vi "AxisWriteRegs.vi"(8 "error in":errorcluster, 10 "AxisWriteValues":T1={"AxisTarget"=0.0, "AxisTargetVel"=1.0, "AxisStartReq"=FALSE, "AxisStopReq"=FALSE, "AxisClearReq"=FALSE, "AxisMovetype"=FALSE, "AxisMotorON"=FALSE, "MoveModeControl"=0, "AxisHomingVel"=1.0, "AxisAccDecc"=30.0} {"MoveModeControl" items=["Absolute"=1, "Relative"=2, "Velocity"=3, "Homing"=4, "none"=0]}, 11 "Modbus master":refnum<class "Modbus Master.lvclass">) -> (0 "error out":errorcluster)   [LabVIEW 2020, in "SMCD14_lib.lvlib"]
uses:
  SMCD14_lib.lvlib
  <vilib>/Modbus/master/Modbus Master.lvclass
  AxisWriteValues_typedef.ctl
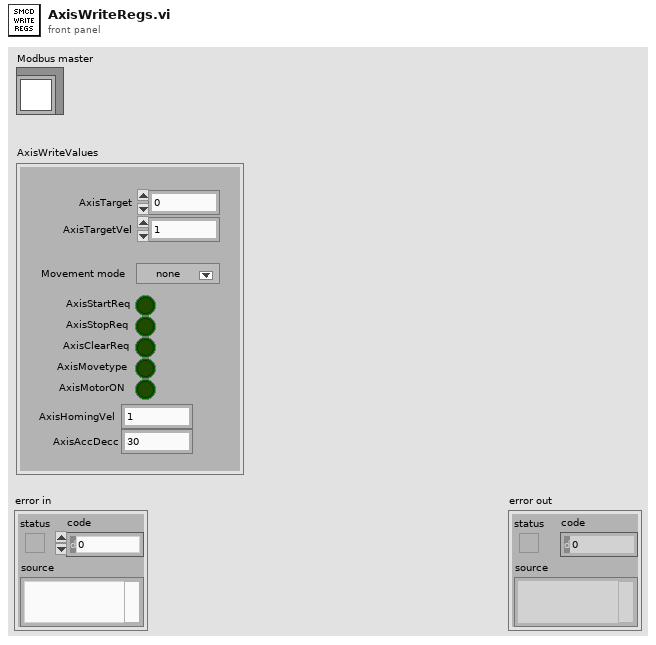
[diagram p1: front panel]
types:
  T1 = typedef "SMCD14_lib.lvlib/AxisWriteValues_typedef.ctl" = cluster{"AxisTarget":dbl, "AxisTargetVel":dbl, "AxisStartReq":bool, "AxisStopReq":bool, "AxisClearReq":bool, "AxisMovetype":bool, "AxisMotorON":bool, "MoveModeControl":u16, "AxisHomingVel":dbl, "AxisAccDecc":dbl}
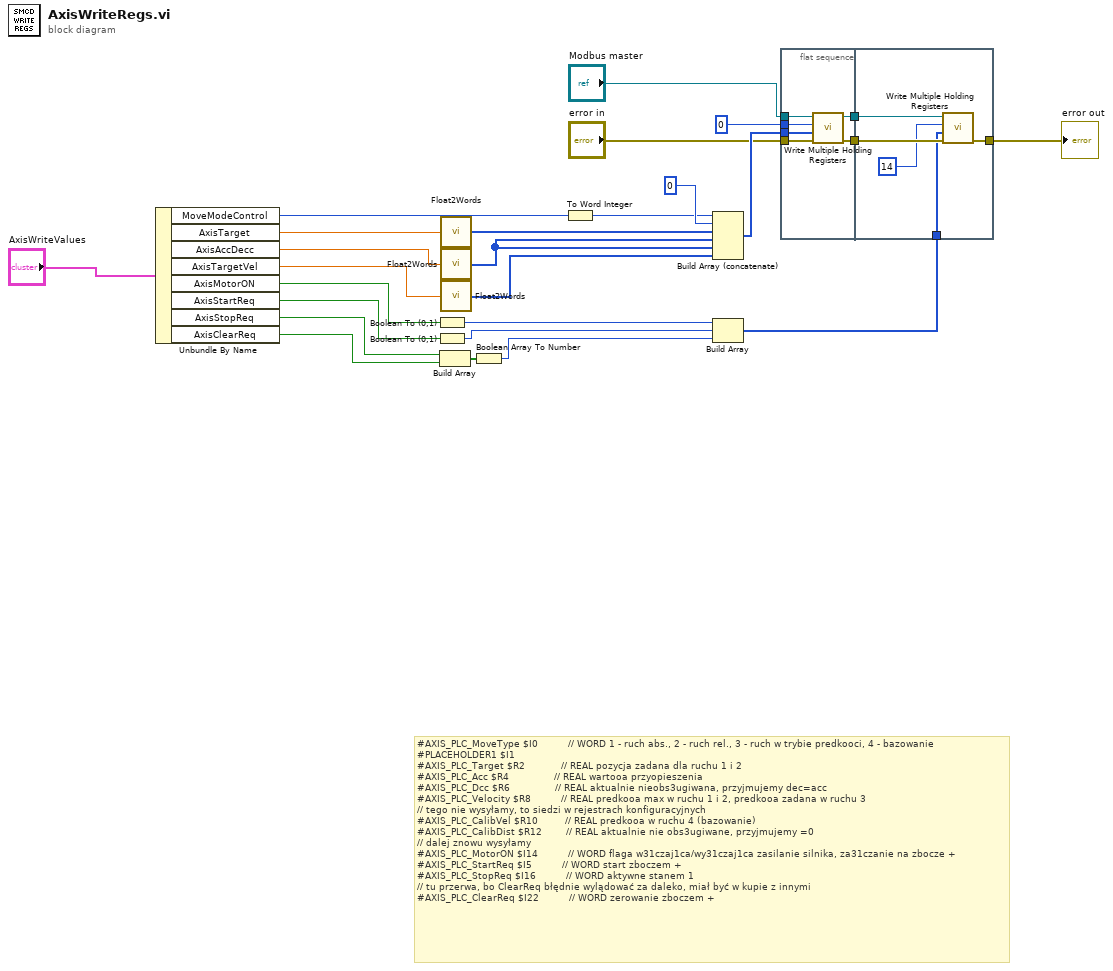
[diagram p0: block diagram]
diagram:
  # "#AXIS_PLC_MoveType $I0          // WORD 1 - ruch abs., 2 - ruch rel., 3 - ruch w trybie predkooci, 4 - bazowanie\n#PLACEHOLDER1 $I1\n#AXIS_PLC_Target $R2            // REAL pozycja zadana dla ruchu 1 i 2\n#AXIS_PLC_Acc $R4               // REAL wartooa przyopieszenia\n#AXIS_PLC_Dcc $R6               // REAL aktualnie nieobs3ugiwana, przyjmujemy dec=acc\n#AXIS_PLC_Velocity $R8          // REAL predkooa max w ruchu 1 i 2, predkooa zadana w ruchu 3\n// tego nie wysyłamy, to siedzi w rejestrach konfiguracyjnych\n#AXIS_PLC_CalibVel $R10         // REAL predkooa w ruchu 4 (bazowanie)\n#AXIS_PLC_CalibDist $R12        // REAL aktualnie nie obs3ugiwane, przyjmujemy =0\n// dalej znowu wysyłamy\n#AXIS_PLC_MotorON $I14          // WORD flaga w31czaj1ca/wy31czaj1ca zasilanie silnika, za31czanie na zbocze +\n#AXIS_PLC_StartReq $I5          // WORD start zboczem +\n#AXIS_PLC_StopReq $I16          // WORD aktywne stanem 1\n// tu przerwa, bo ClearReq błędnie wylądować za daleko, miał być w kupie z innymi\n#AXIS_PLC_ClearReq $I22          // WORD zerowanie zboczem +"
  n1 = Unbundle By Name("AxisWriteValues") -> ("MoveModeControl"=w15:u16, "AxisTarget"=w17:dbl, "AxisAccDecc"=w13:dbl, "AxisTargetVel"=w11:dbl, "AxisMotorON"=w9:bool, "AxisStartReq"=w7:bool, "AxisStopReq"=w3:bool, "AxisClearReq"=w4:bool)
  n2 = Boolean To (0,1)(Boolean=w9) -> (0, 1=w8:i16)
  n3 = Boolean To (0,1)(Boolean=w7) -> (0, 1=w6:i16)
  n4 = Build Array(w3, w4) -> (w2:bool[])
  n5 = call "Float2Words.vi"("value"=w17) -> ("output"=w16:u16[])  [unwired: 4 in]
  n6 = call "Float2Words.vi"("value"=w13) -> ("output"=w12:u16[])  [unwired: 4 in]
  n7 = call "Float2Words.vi"("value"=w11) -> ("output"=w10:u16[])  [unwired: 4 in]
  n8 = Boolean Array To Number(Boolean array=w2) -> (number=w1:u32)
  n9 = To Word Integer(number=w15) -> (16bit integer=w14:i16)
  n10 = Build Array (concatenate)(w14, u16 0 ("element"), w16, w12, w12, w10) -> (w24:u16[])
  n11 = Build Array(w8, w6, w1) -> (w5:u32[])
  n12 = flat-sequence {
    tunnel: [w32] -> w21
    tunnel: [w31] -> w20
    tunnel: "error in" -> [w28]
    tunnel: w24 -> [w29]
    tunnel: u16 0 ("starting address") -> [w27]
    tunnel: "Modbus master" -> [w30]
    tunnel: [w37] -> w23
    tunnel: w5 -> [w34]
    tunnel: w20 -> [w35]
    tunnel: w21 -> [w36]
    frame #0 {
      n13 = call-dynamic "Write Multiple Holding Registers.vi"("error in (no error)"=w28, "holding register values"=w29, "starting address"=w27, "Modbus master in"=w30) -> ("error out"=w32:errorcluster, "Modbus master out"=w31:refnum<class "Modbus Master.lvclass">)  [unwired: 6 in]
    }
    frame #1 {
      n14 = call-dynamic "Write Multiple Holding Registers.vi"("error in (no error)"=w36, "holding register values"=w34, "starting address"=u16 14, "Modbus master in"=w35) -> ("error out"=w37:errorcluster)  [unwired: 6 in, 1 out]
    }
  }
  "error out" <- w23
